vi "Main.vi"(8 "error in":errorcluster) -> (0 "error out":errorcluster)   [LabVIEW 2016, in "Trace Grabber.lvlib"]
doc: "(<B>Filename</B>: Actor Framework.lvlib:Actor.lvclass:Actor Core.vi)\n\nReceives messages to the actor, reacts to them, and initiates any error handling that may shut the actor down.\n\nDescendant classes may override this VI to append parallel tasks for the actor to complete while it handles messages. Overrides use the Call Parent Method node."
uses:
  Trace Grabber.lvlib
  Support VIs/Message Queue/Enqueue Message (Single).vi
  Support VIs/Message Queue/Enqueue Message (Multiple).vi
  <vilib>/Utility/error.llb/Error Cluster From Error Code.vi
  <vilib>/ErrorRing/Error Ring.xnode
  Support VIs/Message Queue/Message Queue.lvlib
panel:
  in  "Log":string
  in  "Focus":i32=100 min=100 max=1000 format="%.0f um"
  in  "Path":path
  in  "Lock focus?":bool
  in  "Stage Control":enum32{"Jog", "S-Scan"}(tab)
  in  "X Range":i32=100 min=100 max=1000 format="%.0f um"
  in  "Y Range":i32=100 min=100 max=1000 format="%.0f um"
  in  "Grid Interval":i32=100 min=100 max=1000 format="%.0f um"
  out "Stage Position":cluster{"X":dbl, "Y":dbl}[](graph)
  out "Duration per Period":dbl format="%#_g ms"
  in  "Fixed Scan Parameters":T1 {"Absolute Delay" format="%d ps"}
  in  "Periodic Scan Parameters":T2={"Range"=10, "Offset"=0, "Frequency"=10} {"Frequency" min=5 max=50 step=1 format="%d Hz"; "Offset" format="%d ps"; "Range" min=10 max=150 step=1 format="%d ps"}
  in  "Save Results":bool
  in  "Abort":bool
  in  "Start":bool
  in  "Free Run":bool
  in  "# Repeats":i32=20 min=1 max=65536 step=1
  out "Total Duration":dbl format="%#_g ms"
  in  "Samples per Period":i32=100 min=8 max=768 step=1
  in  "Gate Time":i32(ring)=500 items=["100 us"=100, "200 us"=200, "500 us"=500, "1 ms"=1000, "2 ms"=2000, "5 ms"=5000, "10 ms"=10000]
  in  "Is fixed scan?":bool
  out "Traces":u32[](graph)
  in  "Quit":bool
  # "Periodic Scan"
  # "Fixed Scan"
  # "Photon Counter"
  # "Measurements"
  # "Stage Control"
  # "Operations"
  # "Directly click on the plot to move the stage to new position."
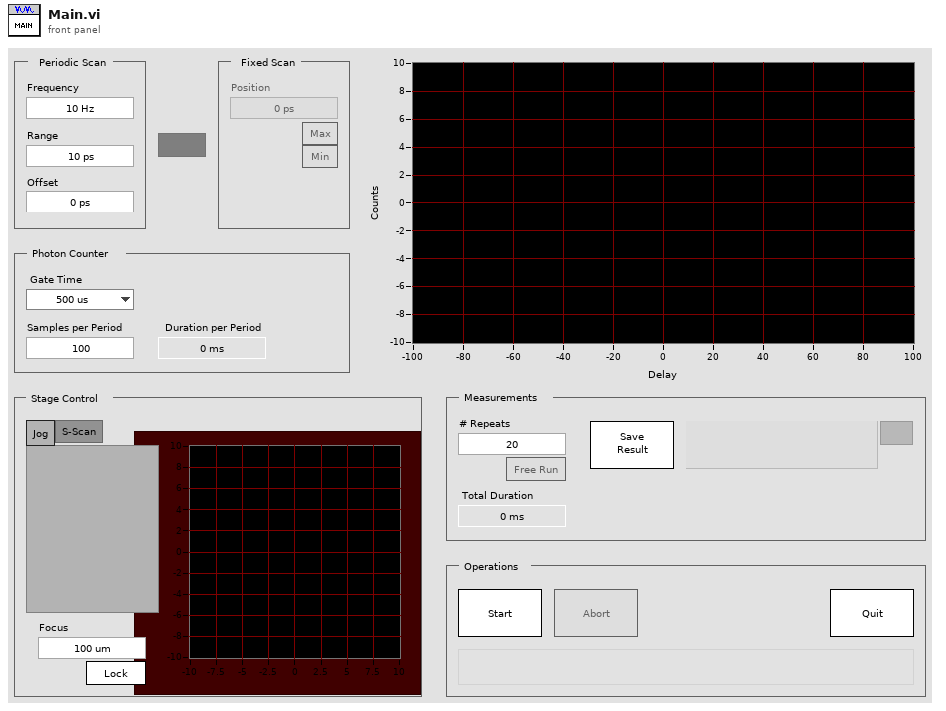
[diagram p1: front panel]
types:
  T1 = cluster{"Absolute Delay":i32, "To Min":bool, "To Max":bool}
  T2 = cluster{"Range":i32, "Offset":i32, "Frequency":i32}
  T3 = typedef "Message Queue.lvlib/Message Queues.ctl" = cluster{"UI":refnum<queue>, "Acquisition":refnum<queue>, "Scanner":refnum<queue>, "Logging":refnum<queue>}
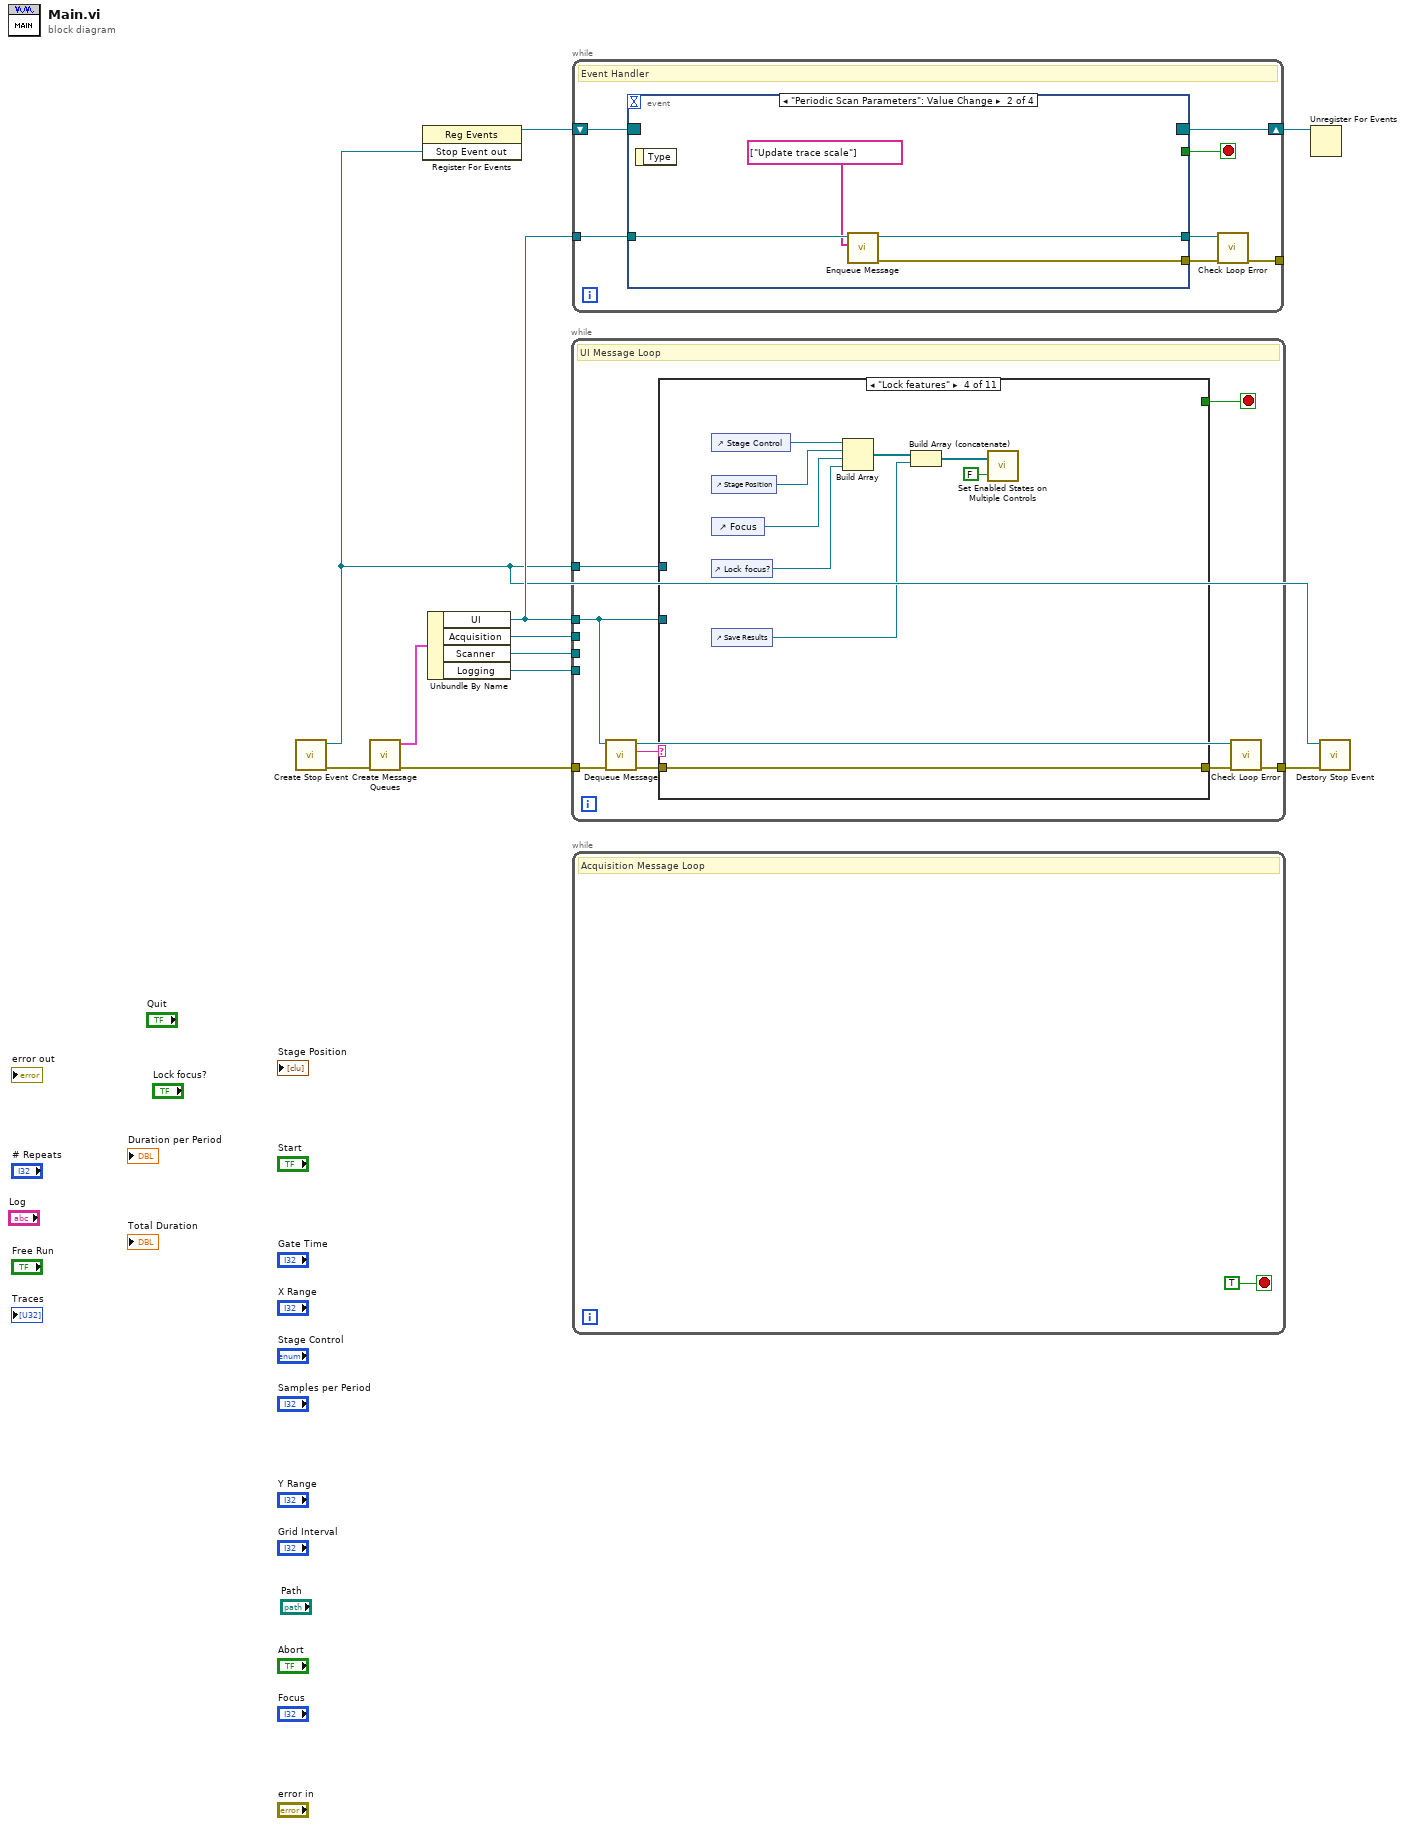
[diagram p0: block diagram]
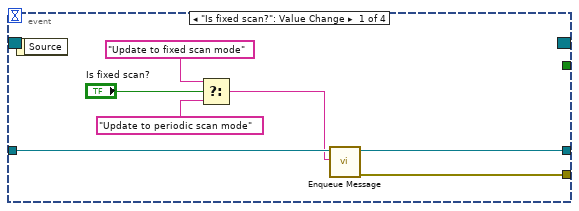
[diagram p2: hidden frame]
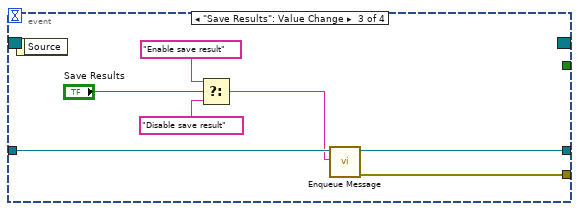
[diagram p3: hidden frame]
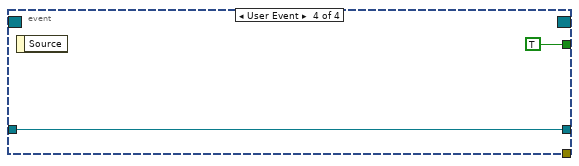
[diagram p4: hidden frame]
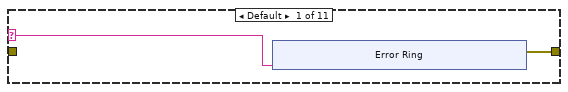
[diagram p5: hidden frame]
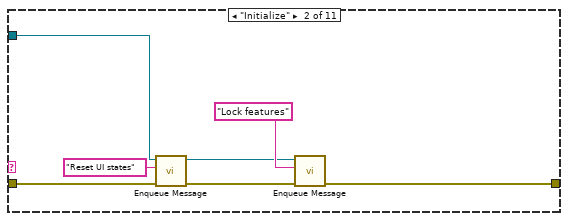
[diagram p6: hidden frame]
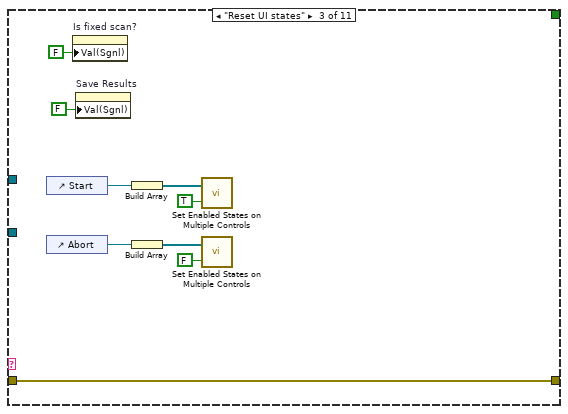
[diagram p7: hidden frame]
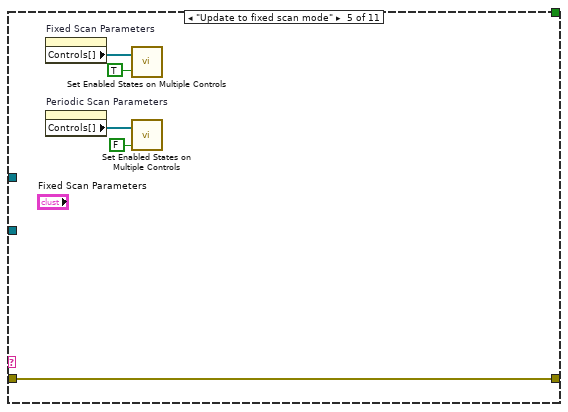
[diagram p8: hidden frame]
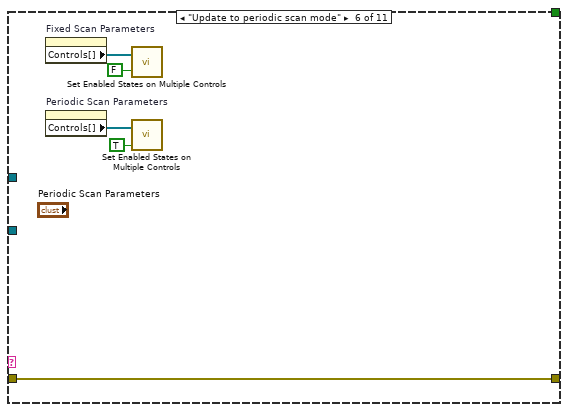
[diagram p9: hidden frame]
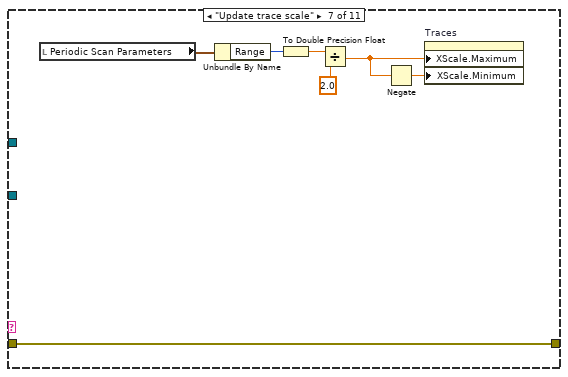
[diagram p10: hidden frame]
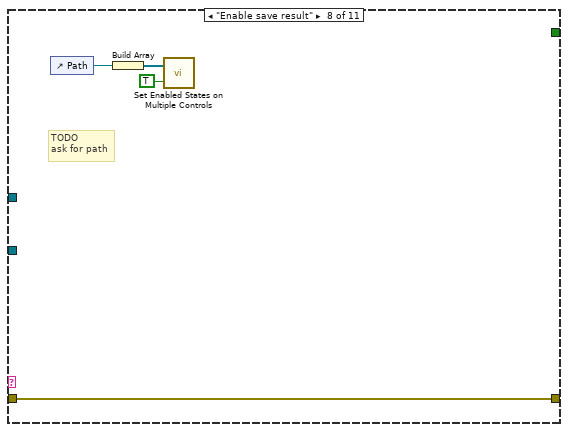
[diagram p11: hidden frame]
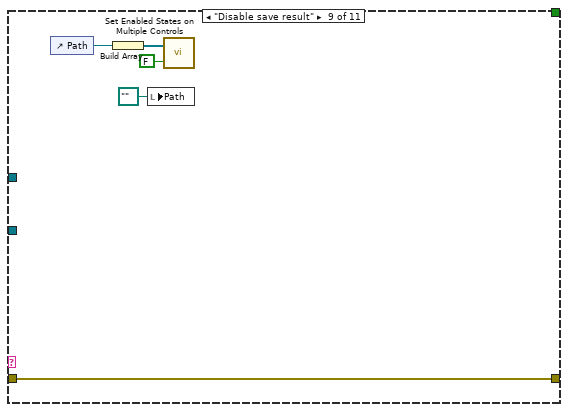
[diagram p12: hidden frame]
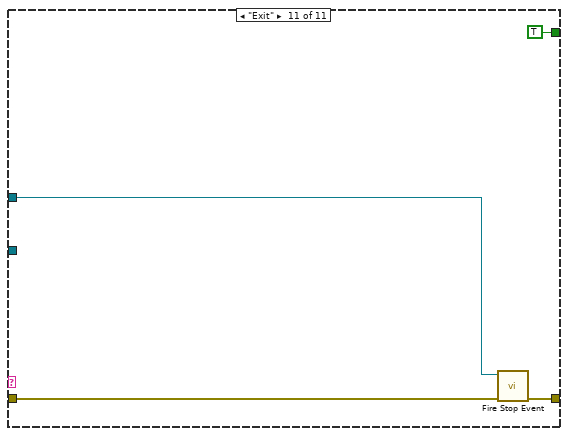
[diagram p14: hidden frame]
diagram:
  n1 = call "Create Stop Event.vi"() -> ("error out"=w5:errorcluster, "Stop Event out"=w1:refnum<user-event>)  [unwired: 10 in]
  n2 = call "Create Message Queues.vi"("error in (no error)"=w5) -> ("error out"=w11:errorcluster, "Message Queues out"=w6:T3)  [unwired: 9 in]
  n3 = register-events(w1) -> (reference out=w4:refnum<event-registration>)  [unwired: 2 in, 1 out]
  n4 = Unbundle By Name(w6) -> ("UI"=w7:refnum<queue>, "Acquisition"=w8:refnum<queue>, "Scanner"=w9:refnum<queue>, "Logging"=w10:refnum<queue>)
  n5 = while {
    tunnel: w11 -> [w20]
    tunnel: w10 -> [_]
    tunnel: w9 -> [_]
    tunnel: w8 -> [_]
    tunnel: w7 -> [w12]
    tunnel: [w16] -> w2
    tunnel: w1 -> [w13]
    stop <- w14 stop-if-true
    # "UI Message Loop"
    n6 = call "Dequeue Message.vi"("error in (no error)"=w20, "Message Queue in"=w12) -> ("error out"=w18:errorcluster, "State"=w19:string, "Message Queue out"=w15:refnum<queue>)  [unwired: 6 in, 1 out]
    n7 = case shown="\"Lock features\"" w19 {
      selector: w19 -> [w22 _ _ _ _ _ _ _ _ _ _]
      tunnel: w18 -> [_ w35 w45 w46 w55 w60 w71 w75 w80 w81 w84]
      tunnel: [w21 w32 w45 w46 w55 w60 w71 w75 w80 w81 w83] -> w17
      tunnel: [_ _ _ _ _ _ _ _ _ _ TRUE] -> w14
      tunnel: w13 -> [_ _ _ _ _ _ _ _ _ _ w85]
      tunnel: w12 -> [_ w36 _ _ _ _ _ _ _ _ _]
      frame Default {
        n8 = xnode "Error Ring"("parameter 0"=w22) -> ("error out"=w21:errorcluster)
      }
      frame "Initialize" {
        n9 = call-poly "Enqueue Message.vi"("error in (no error)"=w35, "State"="Reset UI states", "Message Queue in"=w36) -> ("error out"=w33:errorcluster, "Message Queue out"=w30:refnum<queue>)  [unwired: 7 in]
        n10 = call-poly "Enqueue Message.vi"("error in (no error)"=w33, "State"="Lock features", "Message Queue in"=w30) -> ("error out"=w32:errorcluster)  [unwired: 7 in, 1 out]
      }
      frame "Reset UI states" {
        n11 = control-ref of="Start"() -> (w42:refnum<vi>)
        n12 = control-ref of="Abort"() -> (w40:refnum<vi>)
        n13 = property on="Is fixed scan?" class="Bool (strict)"("Val(Sgnl)"=FALSE ("Value (Signaling)")) -> ()  [unwired: 2 in, 2 out]
        n14 = property on="Save Results" class="Bool (strict)"("Val(Sgnl)"=FALSE ("Value (Signaling)")) -> ()  [unwired: 2 in, 2 out]
        n15 = Build Array(w42) -> (w41:refnum<vi>[])
        n16 = Build Array(w40) -> (w39:refnum<vi>[])
        n17 = call "Set Enabled States on Multiple Controls.vi"("Enable?"=TRUE, "Control Refnums"=w41) -> ()  [unwired: 1 in]
        n18 = call "Set Enabled States on Multiple Controls.vi"("Enable?"=FALSE, "Control Refnums"=w39) -> ()  [unwired: 1 in]
      }
      frame "Lock features" {
        n19 = control-ref of="Stage Control"() -> (w54:refnum<vi>)
        n20 = control-ref of="Stage Position"() -> (w53:refnum<vi>)
        n21 = control-ref of="Focus"() -> (w52:refnum<vi>)
        n22 = control-ref of="Lock focus?"() -> (w51:refnum<vi>)
        n23 = control-ref of="Save Results"() -> (w49:refnum<vi>)
        n24 = Build Array(w54, w53, w52, w51) -> (w50:refnum<vi>[])
        n25 = Build Array (concatenate)(w50, w49) -> (w48:refnum<vi>[])
        n26 = call "Set Enabled States on Multiple Controls.vi"("Enable?"=FALSE, "Control Refnums"=w48) -> ()  [unwired: 1 in]
      }
      frame "Update to fixed scan mode" {
        n27 = property on="Fixed Scan Parameters" class="Clust"() -> ("Controls[]"=w59:refnum<vi>[])  [unwired: 2 in, 2 out]
        n28 = property on="Periodic Scan Parameters" class="Clust (strict)"() -> ("Controls[]"=w57:refnum<vi>[])  [unwired: 2 in, 2 out]
        n29 = call "Set Enabled States on Multiple Controls.vi"("Enable?"=TRUE, "Control Refnums"=w59) -> ()  [unwired: 1 in]
        n30 = call "Set Enabled States on Multiple Controls.vi"("Enable?"=FALSE, "Control Refnums"=w57) -> ()  [unwired: 1 in]
      }
      frame "Update to periodic scan mode" {
        n31 = property on="Fixed Scan Parameters" class="Clust"() -> ("Controls[]"=w64:refnum<vi>[])  [unwired: 2 in, 2 out]
        n32 = property on="Periodic Scan Parameters" class="Clust (strict)"() -> ("Controls[]"=w62:refnum<vi>[])  [unwired: 2 in, 2 out]
        n33 = call "Set Enabled States on Multiple Controls.vi"("Enable?"=FALSE, "Control Refnums"=w64) -> ()  [unwired: 1 in]
        n34 = call "Set Enabled States on Multiple Controls.vi"("Enable?"=TRUE, "Control Refnums"=w62) -> ()  [unwired: 1 in]
      }
      frame "Update trace scale" {
        n35 = local read "Periodic Scan Parameters"() -> (w70:T2)
        n36 = Unbundle By Name(w70) -> ("Range"=w69:i32)
        n37 = To Double Precision Float(number=w69) -> (double precision float=w65:dbl)
        n38 = Divide(x=w65, y=2.0) -> (x/y=w66:dbl)
        n39 = Negate(x=w66) -> (-x=w67:dbl)
        n40 = property on="Traces" class="WFGraph (strict)"("XScale.Maximum"=w66, "XScale.Minimum"=w67) -> ()  [unwired: 2 in, 2 out]
      }
      frame "Enable save result" {
        # "TODO\nask for path"
        n41 = control-ref of="Path"() -> (w74:refnum<vi>)
        n42 = Build Array(w74) -> (w73:refnum<vi>[])
        n43 = call "Set Enabled States on Multiple Controls.vi"("Enable?"=TRUE, "Control Refnums"=w73) -> ()  [unwired: 1 in]
      }
      frame "Disable save result" {
        n44 = control-ref of="Path"() -> (w79:refnum<vi>)
        n45 = Build Array(w79) -> (w78:refnum<vi>[])
        n46 = local write "Path"(path "" ("Path")) -> ()
        n47 = call "Set Enabled States on Multiple Controls.vi"("Enable?"=FALSE, "Control Refnums"=w78) -> ()  [unwired: 1 in]
      }
      frame "Error" {
      }
      frame "Exit" {
        n48 = call "Fire Stop Event.vi"("error in (no error)"=w84, "Stop Event in"=w85) -> ("error out"=w83:errorcluster)  [unwired: 9 in]
      }
    }
    n49 = call "Check Loop Error.vi"("error in (no error)"=w17, "Message Queue in"=w15) -> ("error out"=w16:errorcluster)  [unwired: 7 in, 2 out]
  }
  n50 = while {
    tunnel: w7 -> [w92]
    tunnel: [w90] -> _
    shift-right: [w87] -> w3
    shift-left: w4 -> [w89]
    stop <- w88 stop-if-true
    # "Event Handler"
    n51 = event shown="[1] \"Periodic Scan Parameters\": Value Change" {
      selector: w89 -> [_ _ _ _]
      dyn-events: [_ _ _ _] -> w87
      timeout: _ -> [_ _ _ _]
      tunnel: w92 -> [w99 w103 w110 w111]
      tunnel: [w98 w102 w109 _] -> w91
      tunnel: [_ _ _ TRUE] -> w88
      tunnel: [w93 w101 w104 w111] -> w86
      event "Is fixed scan?": Value Change {
        n52 = event-data() -> ()  [unwired: 1 in, 1 out]
        n53 = Select(t="Update to fixed scan mode" ("State"), s="Is fixed scan?", f="Update to periodic scan mode" ("State")) -> (s? t:f=w94:string)
        n54 = call-poly "Enqueue Message.vi"("State"=w94, "Message Queue in"=w99) -> ("error out"=w98:errorcluster, "Message Queue out"=w93:refnum<queue>)  [unwired: 8 in]
      }
      event "Periodic Scan Parameters": Value Change {
        n55 = event-data() -> ()  [unwired: 1 in, 1 out]
        n56 = call-poly "Enqueue Message.vi"("States"=string[] ["Update trace scale"], "Message Queue in"=w103) -> ("error out"=w102:errorcluster, "Message Queue out"=w101:refnum<queue>)  [unwired: 8 in]
      }
      event "Save Results": Value Change {
        n57 = event-data() -> ()  [unwired: 1 in, 1 out]
        n58 = Select(t="Enable save result" ("State"), s="Save Results", f="Disable save result" ("State")) -> (s? t:f=w106:string)
        n59 = call-poly "Enqueue Message.vi"("State"=w106, "Message Queue in"=w110) -> ("error out"=w109:errorcluster, "Message Queue out"=w104:refnum<queue>)  [unwired: 8 in]
      }
      event User Event {
        n60 = event-data() -> ()  [unwired: 1 in, 1 out]
      }
    }
    n61 = call "Check Loop Error.vi"("error in (no error)"=w91, "Message Queue in"=w86) -> ("error out"=w90:errorcluster)  [unwired: 7 in, 2 out]
  }
  n62 = while {
    stop <- TRUE stop-if-true
    # "Acquisition Message Loop"
  }
  n63 = Unregister For Events(event registration refnum=w3) -> ()  [unwired: 1 in, 1 out]
  n64 = call "Destory Stop Event.vi"("error in (no error)"=w2, "Stop Event in"=w1) -> ()  [unwired: 9 in, 1 out]
